vi "ADC Read Raw.vi"(8 "error in (no error)":errorcluster, 10 "ADC Channel Selection":T2, 11 "LINX-ADS1X15 in":refnum<class "LINX-ADS1X15.lvclass">) -> (0 "error out":errorcluster, 2 "ADC Raw":i16, 3 "LINX-ADS1X15 out":refnum<class "LINX-ADS1X15.lvclass">)   [LabVIEW 2020, in "LINX-ADS1X15.lvclass"]
uses:
  LINX-ADS1X15.lvclass
  Channel Selection.ctl
  Programmable Gain Selection.ctl
  e8cd9032-853c-4972-a891-994538bc7c31.vi
  LINX I2C/LINX I2C.lvclass
panel:
  out "Numeric":u16 format="%.0x"
  out "result":T1
  out "Boolean array":bool[](array[boolean])
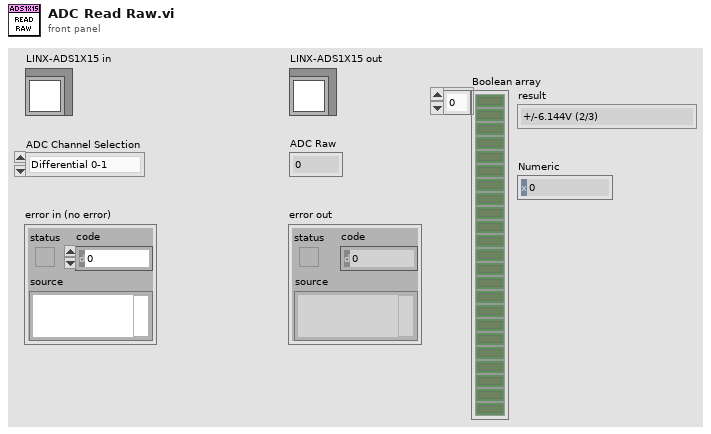
[diagram p1: front panel]
types:
  T1 = typedef "LINX-ADS1X15.lvclass/Programmable Gain Selection.ctl" = enum16{"+/-6.144V (2/3)", "+/-4.096V (1)", "+/-2.048V (2)", "+/-1.024V (4)", "+/-0.512V (8)", "+/-0.256V (16)"}
  T2 = typedef "LINX-ADS1X15.lvclass/Channel Selection.ctl" = enum16{"Differential 0-1", "Differential 2-3", "Single Ended 0", "Single Ended 1", "Single Ended 2", "Single Ended 3"}
  T3 = typedef "LINX-ADS1X15.lvclass/ADC Type Selection.ctl" = enum16{"ADS1015", "ADS1115"}
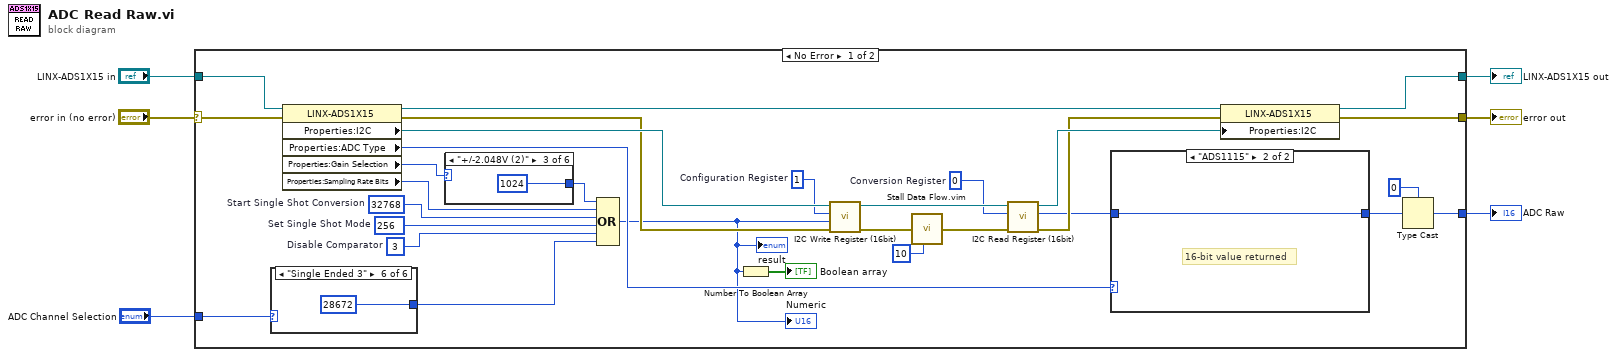
[diagram p0: block diagram]
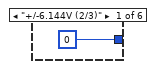
[diagram p2: hidden frame]
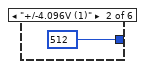
[diagram p3: hidden frame]
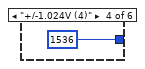
[diagram p4: hidden frame]
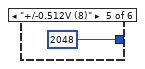
[diagram p5: hidden frame]
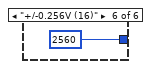
[diagram p6: hidden frame]
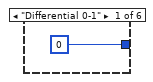
[diagram p7: hidden frame]
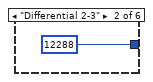
[diagram p8: hidden frame]
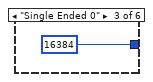
[diagram p9: hidden frame]
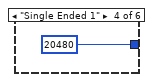
[diagram p10: hidden frame]
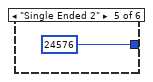
[diagram p11: hidden frame]
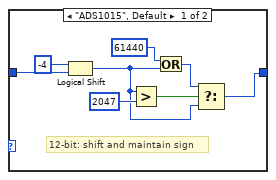
[diagram p12: hidden frame]
diagram:
  n1 = case shown="No Error" "error in (no error)" {
    selector: "error in (no error)" -> [w33 w59]
    tunnel: [w32 w59] -> w5
    tunnel: [w34 w58] -> w3
    tunnel: "LINX-ADS1X15 in" -> [w36 w58]
    tunnel: "ADC Channel Selection" -> [w10 _]
    tunnel: [w21 _] -> w1
    frame No Error {
      w11 = u16 256  # Set Single Shot Mode
      w17 = u16 3  # Disable Comparator
      w16 = u16 32768  # Start Single Shot Conversion
      w25 = u8 0  # Conversion Register
      w26 = u8 1  # Configuration Register
      n2 = case shown="\"Single Ended 3\"" w10 {
        tunnel: [u16 0 u16 12288 u16 16384 u16 20480 u16 24576 u16 28672] -> w9
        frame "Differential 0-1" {
        }
        frame "Differential 2-3" {
        }
        frame "Single Ended 0" {
        }
        frame "Single Ended 1" {
        }
        frame "Single Ended 2" {
        }
        frame "Single Ended 3" {
        }
      }
      n3 = property class="LINX-ADS1X15"(reference=w36, error in=w33) -> (reference out=w35:refnum<class "LINX-ADS1X15.lvclass">, error out=w29:errorcluster, "Properties:I2C"=w30:refnum<class "LINX I2C.lvclass">, "Properties:ADC Type"=w24:T3, "Properties:Gain Selection"=w8:T1, "Properties:Sampling Rate Bits"=w12:u16)
      n4 = case shown="\"+/-2.048V (2)\"" w8 {
        tunnel: [u16 0 u16 512 u16 1024 u16 1536 u16 2048 u16 2560] -> w7
        frame "+/-6.144V (2/3)" {
        }
        frame "+/-4.096V (1)" {
        }
        frame "+/-2.048V (2)" {
        }
        frame "+/-1.024V (4)" {
        }
        frame "+/-0.512V (8)" {
        }
        frame "+/-0.256V (16)" {
        }
      }
      n5 = Compound Arithmetic op=OR(w7, w12, w16, w11, w17, w9) -> (w13:u16)
      "result" <- w13
      "Numeric" <- w13
      n6 = Number To Boolean Array(number=w13) -> (Boolean array=→"Boolean array":bool[])
      n7 = call "I2C Write Register (16bit).vi"("error in (no error)"=w29, "Value"=w13, "Register Address"=w26, "LINX I2C in"=w30) -> ("error out"=w20:errorcluster, "LINX I2C out"=w31:refnum<class "LINX I2C.lvclass">)  [unwired: 6 in]
      n8 = call "Stall Data Flow.vim"("value in"=w20, "milliseconds to wait"=u32 10) -> ("value out"=w19:errorcluster)  [unwired: 1 out]
      n9 = call "I2C Read Register (16bit).vi"("error in (no error)"=w19, "Register Address"=w25, "LINX I2C in"=w31) -> ("error out"=w27:errorcluster, "Value"=w15:u16, "LINX I2C out"=w28:refnum<class "LINX I2C.lvclass">)  [unwired: 6 in]
      n10 = case shown="\"ADS1115\"" w24 {
        tunnel: w15 -> [w56 w57]
        tunnel: [w50 w57] -> w22
        frame "ADS1015", Default {
          # "12-bit: shift and maintain sign"
          n11 = Logical Shift(y=i16 -4, x=w56) -> (x << y=w49:u16)
          n12 = Greater?(x=w49, y=u16 2047) -> (0:w53:bool)
          n13 = Or(x=u16 61440 ("y"), y=w49) -> (x .or. y?=w51:u16)
          n14 = Select(t=w51, s=w53, f=w49) -> (s? t:f=w50:u16)
        }
        frame "ADS1115" {
          # "16-bit value returned"
        }
      }
      n15 = property class="LINX-ADS1X15"(reference=w35, error in=w27, "Properties:I2C"=w28) -> (reference out=w34:refnum<class "LINX-ADS1X15.lvclass">, error out=w32:errorcluster)
      n16 = Type Cast(type=i16 0 ("ADC Raw"), x=w22) -> (*(type *) &x=w21:i16)
    }
    frame Error {
    }
  }
  "error out" <- w5
  "LINX-ADS1X15 out" <- w3
  "ADC Raw" <- w1
